vi "Config GSM Framed.vi"(0 "VISA Resource Name":refnum<visa-resource-name>, 1 "Frame Trigger (2:TRIGGER KEY)":enum16{"BUS", "EXTERNAL", "TRIGGER KEY"}(ring)=enum."TRIGGER KEY", 2 "Ext Delay (F:OFF)":bool, 3 "Ext Delay Bits (0)":i32, 5 "Frame Repeat (F:CONT)":bool, 11 "error in (no error)":errorcluster {"code" format="%.0x"}, 12 "Secondary Frame (F:OFF)":bool, 13 "Sec Frame Trigger (1:EXT)":enum16{"BUS", "EXTERNAL", "TRIGGER KEY"}(ring)=enum."EXTERNAL") -> (4 "VISA Resource Name Out":refnum<visa-resource-name>, 15 "error out":errorcluster {"code" format="%.0x"})   [LabVIEW 2012, in "Agilent ESG Series.lvlib"]
doc: "This VI is used to configure NADC framed data.\nRun the Config NADC framed Timeslot.vi after this vi to configure an individual Timeslot."
uses:
  <instrlib>/Agilent ESG Series/Agilent ESG Series.lvlib
panel:
  # "SINGLE"
  # "CONT"
  # "ON"
  # "OFF"
  # "ON"
  # "OFF"
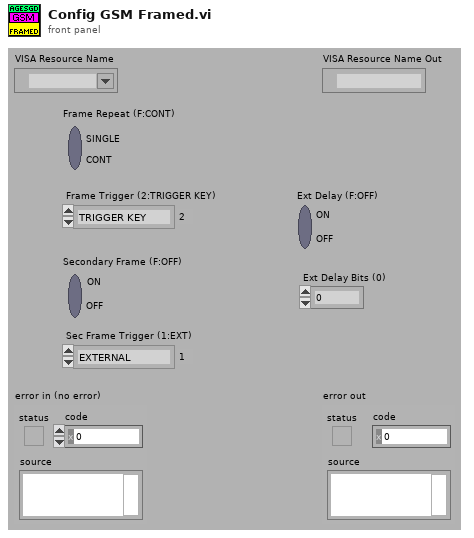
[diagram p1: front panel]
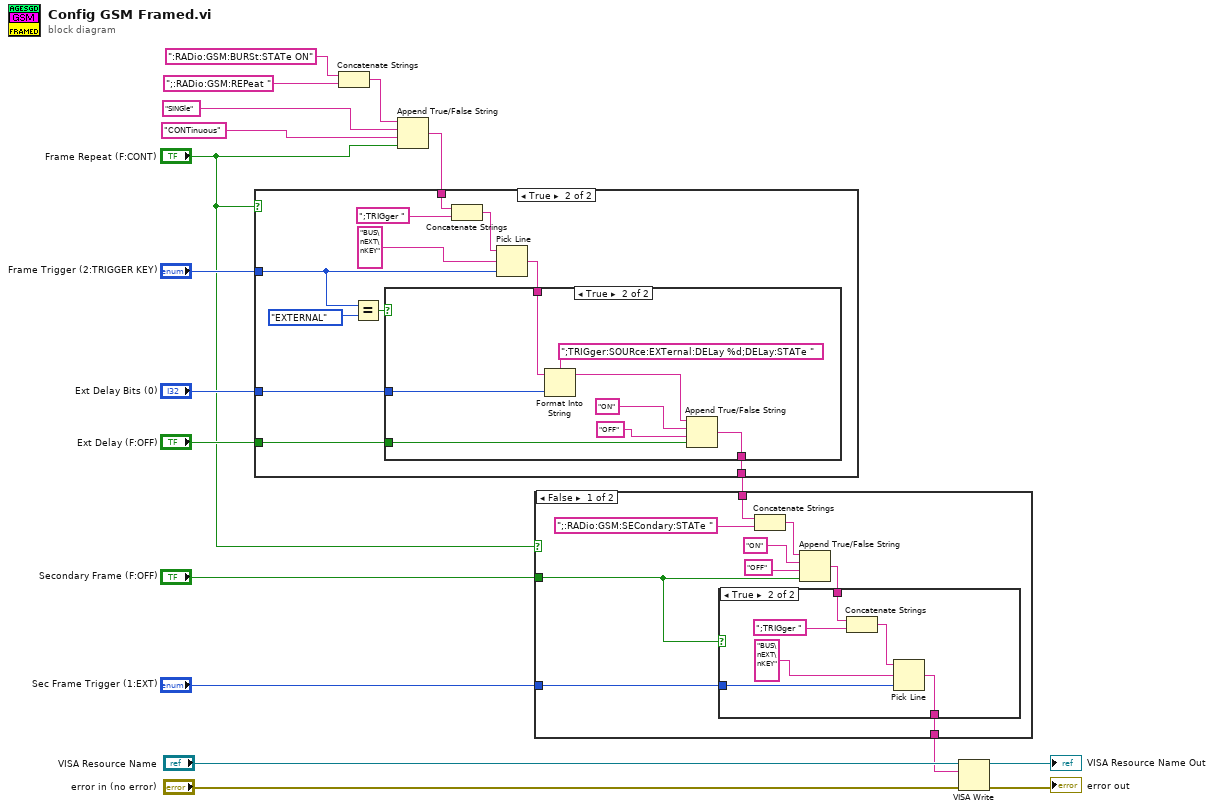
[diagram p0: block diagram]
diagram:
  n1 = Concatenate Strings(":RADio:GSM:BURSt:STATe ON", ";:RADio:GSM:REPeat ") -> (w12:string)
  n2 = Append True/False String(1:"Frame Repeat (F:CONT)", 2:"CONTinuous" ("false string"), 3:"SINGle" ("true string"), 4:w12) -> (0:w2:string)
  n3 = case shown="True" "Frame Repeat (F:CONT)" {
    tunnel: w2 -> [w19 w28]
    tunnel: [w19 w23] -> w7
    tunnel: "Frame Trigger (2:TRIGGER KEY)" -> [_ w20]
    tunnel: "Ext Delay Bits (0)" -> [_ w22]
    tunnel: "Ext Delay (F:OFF)" -> [_ w21]
    frame False {
    }
    frame True {
      n4 = Equal?(x=w20, y=enum16{"BUS", "EXTERNAL", "TRIGGER KEY"}."EXTERNAL") -> (x = y?=w24:bool)
      n5 = Concatenate Strings(w28, ";TRIGger ") -> (w27:string)
      n6 = Pick Line(string ("")=w27, multi-line string="BUS\nEXT\nKEY", line index=w20) -> (output string=w26:string)
      n7 = case shown="True" w24 {
        tunnel: w26 -> [w31 w36]
        tunnel: [w31 w34] -> w23
        tunnel: w22 -> [_ w33]
        tunnel: w21 -> [_ w32]
        frame False {
        }
        frame True {
          n8 = Format Into String(format string=";TRIGger:SOURce:EXTernal:DELay %d;DELay:STATe ", initial string=w36, w33) -> (resulting string=w35:string)  [unwired: 1 in, 1 out]
          n9 = Append True/False String(1:w32, 2:"OFF" ("false string"), 3:"ON" ("true string"), 4:w35) -> (0:w34:string)
        }
      }
    }
  }
  n10 = case shown="False" "Frame Repeat (F:CONT)" {
    tunnel: [w48 w56] -> w4
    tunnel: "Secondary Frame (F:OFF)" -> [w47 _]
    tunnel: "Sec Frame Trigger (1:EXT)" -> [w46 _]
    tunnel: w7 -> [w45 w56]
    frame False {
      n11 = Concatenate Strings(w45, ";:RADio:GSM:SECondary:STATe ") -> (w42:string)
      n12 = Append True/False String(1:w47, 2:"OFF" ("false string"), 3:"ON" ("true string"), 4:w42) -> (0:w43:string)
      n13 = case shown="True" w47 {
        tunnel: w43 -> [w49 w52]
        tunnel: [w49 w51] -> w48
        tunnel: w46 -> [_ w50]
        frame False {
        }
        frame True {
          n14 = Concatenate Strings(w52, ";TRIGger ") -> (w55:string)
          n15 = Pick Line(string ("")=w55, multi-line string="BUS\nEXT\nKEY", line index=w50) -> (output string=w51:string)
        }
      }
    }
    frame True {
    }
  }
  n16 = VISA Write(VISA resource name="VISA Resource Name", write buffer=w4, error in (no error)="error in (no error)") -> (VISA resource name out=→"VISA Resource Name Out":refnum<visa-resource-name>, error out=→"error out":errorcluster)  [unwired: 1 out]
